vi "Init Events.vi"(8 "error in (no error)":errorcluster, 11 "Engine in":refnum<class "Engine.lvclass">) -> (0 "error out":errorcluster, 3 "Engine out":refnum<class "Engine.lvclass">)   [LabVIEW 2020, in "TSnax.lvlib" / "Engine.lvclass"]
uses:
  Engine.lvclass
  Open SequenceFile Request.ctl
  SequenceFile/File Load Options.ctl
  SequenceFile/SequenceFile.lvclass
  SequenceFile Response.ctl
  VariableContainer Request.ctl
  VariableContainer Type.ctl
  PropertyObject/PropertyObject.lvclass
  VariableContainer Response.ctl
  New Execution Request.ctl
  Execution/Execution Options.ctl
  Execution Response.ctl
  Execution/Execution.lvclass
  Execution Report Request.ctl
  Report Response.ctl
  Report/Report.lvclass
  Engine.lvclass/Engine.ctl
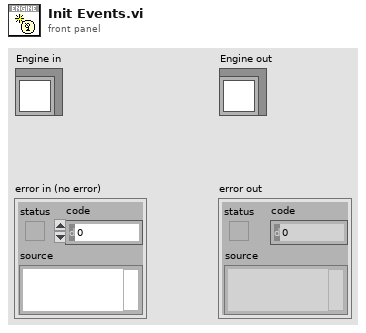
[diagram p1: front panel]
types:
  T1 = typedef "TSnax.lvlib/Engine.lvclass/Execution Report Request.ctl" = cluster{"Execution":refnum<class "Execution.lvclass">, "Notifier":refnum<notifier>}
  T2 = typedef "TSnax.lvlib/Engine.lvclass/New Execution Request.ctl" = cluster{"Options":T3, "Notifier":refnum<notifier>}
  T3 = typedef "TSnax.lvlib/Execution.lvclass/Execution Options.ctl" = cluster{"Use Default Model":bool, "Release Related References":bool}
  T4 = typedef "TSnax.lvlib/Engine.lvclass/VariableContainer Request.ctl" = cluster{"Type":T5, "Scope":refnum<class "PropertyObject.lvclass">, "Lookup String":string, "Notifier":refnum<notifier>}
  T5 = typedef "TSnax.lvlib/Engine.lvclass/VariableContainer Type.ctl" = enum16{"StationGlobals", "TemporaryGlobals", "NewPropertyObject", "SubProperty"}
  T6 = typedef "TSnax.lvlib/Engine.lvclass/Open SequenceFile Request.ctl" = cluster{"File Path":path, "File Load Options":T7, "Current SeqFile":refnum<class "SequenceFile.lvclass">, "Notifier":refnum<notifier>}
  T7 = typedef "TSnax.lvlib/SequenceFile.lvclass/File Load Options.ctl" = cluster{"Use Search Dirs? (T)":bool, "Conflict as Error? (T)":bool, "Check Station Model? (F)":bool, "Preload Modules? (T)":bool, "Skip Load Callback? (F)":bool, "Reload if Loaded? (F)":bool}
  T8 = typedef "TSnax.lvlib/Engine.lvclass/Incoming Events.ctl" = cluster{"Stop Daemon":refnum<user-event>, "Debug Line":refnum<user-event>, "Open SequenceFile":refnum<user-event>, "PropertyObject":refnum<user-event>, "New Execution":refnum<user-event>, "Execution Report":refnum<user-event>}
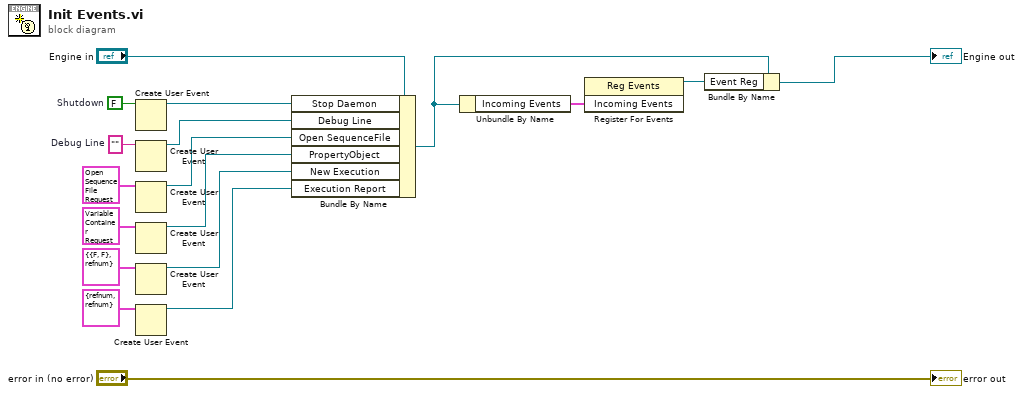
[diagram p0: block diagram]
diagram:
  w10 = ""  # Debug Line
  w16 = FALSE  # Shutdown
  n1 = Create User Event(user event datatype=w16) -> (user event=w15:refnum<user-event>)  [unwired: 1 in, 1 out]
  n2 = Create User Event(user event datatype=w10) -> (user event=w9:refnum<user-event>)  [unwired: 1 in, 1 out]
  n3 = Create User Event(user event datatype=T6 {"File Path"=path "", "File Load Options"={"Use Search Dirs? (T)"=TRUE, "Conflict as Error? (T)"=TRUE, "Check Station Model? (F)"=FALSE, "Preload Modules? (T)"=TRUE, "Skip Load Callback? (F)"=FALSE, "Reload if Loaded? (F)"=FALSE}, "Current SeqFile"=refnum, "Notifier"=refnum} ("Open SequenceFile Request")) -> (user event=w7:refnum<user-event>)  [unwired: 1 in, 1 out]
  n4 = Create User Event(user event datatype=T4 {"Type"=enum."StationGlobals", "Scope"=refnum, "Lookup String"="", "Notifier"=refnum} ("VariableContainer Request")) -> (user event=w5:refnum<user-event>)  [unwired: 1 in, 1 out]
  n5 = Create User Event(user event datatype=T2 {"Options"={"Use Default Model"=FALSE, "Release Related References"=FALSE}, "Notifier"=refnum} ("New Execution Request")) -> (user event=w3:refnum<user-event>)  [unwired: 1 in, 1 out]
  n6 = Create User Event(user event datatype=T1 {"Execution"=refnum, "Notifier"=refnum} ("Execution Report Request")) -> (user event=w1:refnum<user-event>)  [unwired: 1 in, 1 out]
  n7 = Bundle By Name(cluster="Engine in", "Stop Daemon"=w15, "Debug Line"=w9, "Open SequenceFile"=w7, "PropertyObject"=w5, "New Execution"=w3, "Execution Report"=w1) -> (w14:refnum<class "Engine.lvclass">)
  n8 = Unbundle By Name(w14) -> ("Incoming Events"=w13:T8)
  n9 = register-events(w13) -> (reference out=w11:refnum<event-registration>)  [unwired: 2 in, 1 out]
  n10 = Bundle By Name(cluster=w14, "Event Reg"=w11) -> (→"Engine out":refnum<class "Engine.lvclass">)
  "error out" <- "error in (no error)"
